vi "Spectral parameters changed.vi"(9 "Old PSDs":cluster{"f0":dbl, "df":dbl, "magnitude":dbl[]}[](array[cluster]) {"magnitude" format="%.2p"; "f0" format="%.2p"; "df" format="%.2p"}, 10 "New PSDs":cluster{"f0":dbl, "df":dbl, "magnitude":dbl[]}[](array[cluster]) {"magnitude" format="%.2p"; "f0" format="%.2p"; "df" format="%.2p"}) -> (1 "Spectral parameters changed":bool)   [LabVIEW 2020]
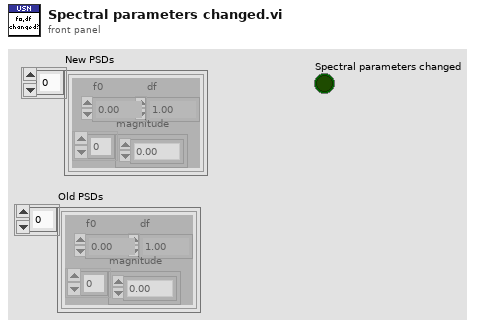
[diagram p1: front panel]
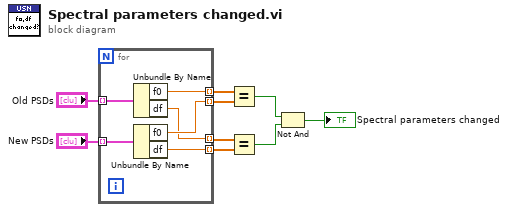
[diagram p0: block diagram]
diagram:
  n1 = for {
    tunnel: "Old PSDs" -> [w15] mode=indexing
    tunnel: [w14] -> w7 mode=indexing
    tunnel: [w11] -> w6 mode=indexing
    tunnel: "New PSDs" -> [w13] mode=indexing
    tunnel: [w10] -> w4 mode=indexing
    tunnel: [w12] -> w5 mode=indexing
    n2 = Unbundle By Name(w15) -> ("f0"=w14:dbl, "df"=w10:dbl)
    n3 = Unbundle By Name(w13) -> ("f0"=w11:dbl, "df"=w12:dbl)
  }
  n4 = Equal?(x=w7, y=w6) -> (x = y?=w3:bool)
  n5 = Equal?(x=w4, y=w5) -> (x = y?=w2:bool)
  n6 = Not And(1:w2, 2:w3) -> (0:→"Spectral parameters changed":bool)
